vi "Relay control.vi"(8 "error in (no error) 2":errorcluster, 10 "outputValues":u16[](array[ring])=[0] items=["low"=0, "high"=1, "Unchange"=255], 11 "gpioDir":enum8{"Output", "Input", "Unchange"}[](array[ring])=[enum."Output"]) -> (0 "error out":errorcluster)   [LabVIEW 2020]
uses:
  mcp2221_dll_um_x64.dll
panel:
  out "handle out":u64=66020
  out "noOfDevs out":u32=1
  in  "WhichToSet":u8(ring)=1 items=["Flash", "SRAM"]
  in  "GPIO Configuration":T1
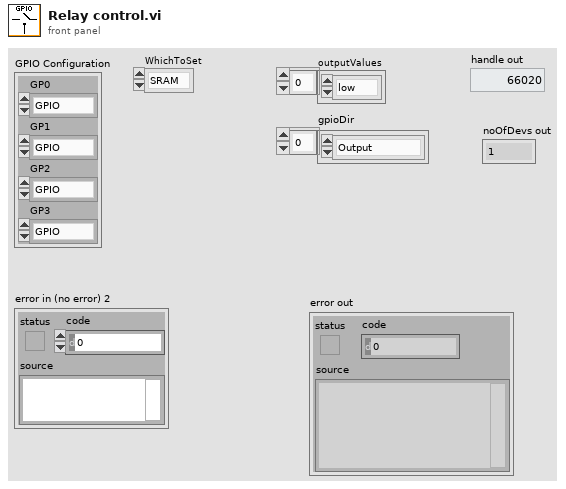
[diagram p1: front panel]
types:
  T1 = cluster{"GP0":enum8{"GPIO", "SSPND", "LED UART RX", "LED UART TX"}, "GP1":enum8{"GPIO", "Clock Out", "ADC1", "DAC1", "Interrupt detection"}, "GP2":enum8{"GPIO", "USBCFG", "ADC2", "DAC2"}, "GP3":enum8{"GPIO", "LED I2C", "ADC3"}}
  T2 = enum8{"GPIO", "SSPND", "LED UART RX", "LED UART TX"}
  T3 = enum8{"GPIO", "Clock Out", "ADC1", "DAC1", "Interrupt detection"}
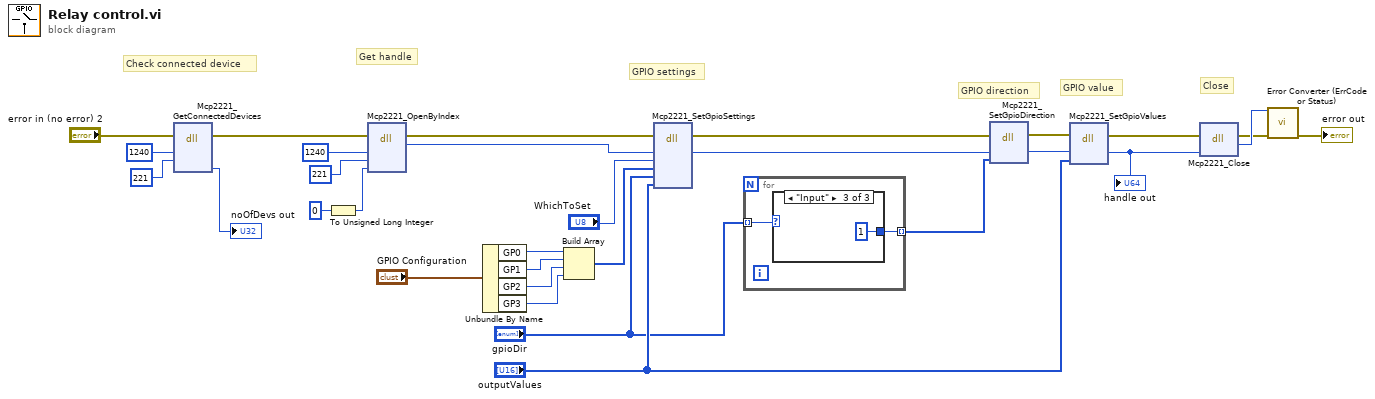
[diagram p0: block diagram]
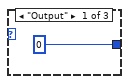
[diagram p2: hidden frame]
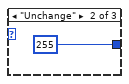
[diagram p3: hidden frame]
diagram:
  # "Close"
  # "GPIO value"
  # "GPIO direction"
  # "GPIO settings"
  # "Get handle"
  # "Check connected device"
  n1 = dll-call lib="C:/Users/tuguialexand/Desktop/Licenta/MCP2221A LabVIEW library/Microchip MCP2221A_64bit/VIs/Private/mcp2221_dll_um_x64.dll" fn="Mcp2221_GetConnectedDevices"(error in="error in (no error) 2", "vid"=u32 1240, "pid"=u32 221) -> (error out=w14:errorcluster, "noOfDevs"=→"noOfDevs out":u32)  [unwired: 6 in, 1 out]
  n2 = To Unsigned Long Integer(number=0 ("index")) -> (unsigned 32bit integer=w17:u32)
  n3 = dll-call lib="C:/Users/tuguialexand/Desktop/Licenta/MCP2221A LabVIEW library/Microchip MCP2221A_64bit/VIs/Private/mcp2221_dll_um_x64.dll" fn="Mcp2221_OpenByIndex"(error in=w14, "VID"=u32 1240, "PID"=u32 221, "index"=w17) -> (error out=w11:errorcluster, "return type"=w8:u64)  [unwired: 5 in, 1 out]
  n4 = Unbundle By Name("GPIO Configuration") -> ("GP0"=w29:T2, "GP1"=w28:T3, "GP2"=w27:enum8{"GPIO", "USBCFG", "ADC2", "DAC2"}, "GP3"=w26:enum8{"GPIO", "LED I2C", "ADC3"})
  n5 = Build Array(w29, w28, w27, w26) -> (w25:u8[])
  n6 = dll-call lib="C:/Users/tuguialexand/Desktop/Licenta/MCP2221A LabVIEW library/Microchip MCP2221A_64bit/VIs/Private/mcp2221_dll_um_x64.dll" fn="Mcp2221_SetGpioSettings"(error in=w11, "handle"=w8, "whichToSet"="WhichToSet", "pinFunctions"=w25, "pinDirections"="gpioDir", "outputValues"="outputValues") -> (error out=w6:errorcluster, "handle"=w4:u64)  [unwired: 7 in, 1 out]
  n7 = for {
    tunnel: "gpioDir" -> [w32] mode=indexing
    tunnel: [w31] -> w7 mode=indexing
    n8 = case shown="\"Input\"" w32 {
      tunnel: [u8 0 u8 255 u8 1] -> w31
      frame "Output" {
      }
      frame "Unchange" {
      }
      frame "Input" {
      }
    }
  }
  n9 = dll-call lib="C:/Users/tuguialexand/Desktop/Licenta/MCP2221A LabVIEW library/Microchip MCP2221A_64bit/VIs/Private/mcp2221_dll_um_x64.dll" fn="Mcp2221_SetGpioDirection"(error in=w6, "handle"=w4, "gpioDir"=w7) -> (error out=w5:errorcluster, "handle"=w3:u64)  [unwired: 4 in, 1 out]
  n10 = dll-call lib="C:/Users/tuguialexand/Desktop/Licenta/MCP2221A LabVIEW library/Microchip MCP2221A_64bit/VIs/Private/mcp2221_dll_um_x64.dll" fn="Mcp2221_SetGpioValues"(error in=w5, "handle"=w3, "gpioValues"="outputValues") -> (error out=w10:errorcluster, "handle"=w9:u64)  [unwired: 4 in, 1 out]
  "handle out" <- w9
  n11 = dll-call lib="C:/Users/tuguialexand/Desktop/Licenta/MCP2221A LabVIEW library/Microchip MCP2221A_64bit/VIs/Private/mcp2221_dll_um_x64.dll" fn="Mcp2221_Close"(error in=w10, "handle"=w9) -> (error out=w12:errorcluster, "return type"=w13:i32)  [unwired: 3 in, 1 out]
  n12 = call "Error Converter (ErrCode or Status).vi"("error code"=w13, "error in (no error)"=w12) -> ("error out"=→"error out":errorcluster)  [unwired: 13 in]
